vi "Test Timed Door API.vi"() -> ()   [LabVIEW 2018]
uses:
  Timed Door.lvclass
  Door/Door.lvclass
  Timed Door.lvclass/Timed Door.ctl
  Set Door.vi
  Set Target Time (seconds).vi
panel:
  out "error out":errorcluster
  in  "Timed Door Target Time (seconds)":dbl=5.0
  in  "Door Switch":enum32{"Open Door", "Close Door"}(radio)=enum."Close Door"
  out "Door":u16(ring)
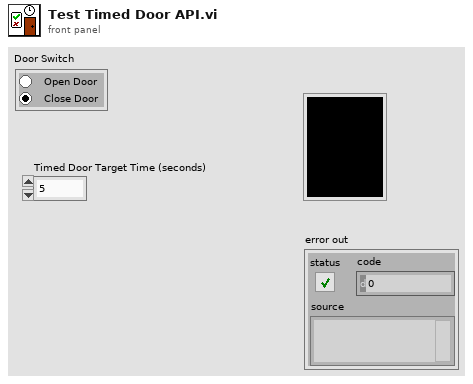
[diagram p1: front panel]
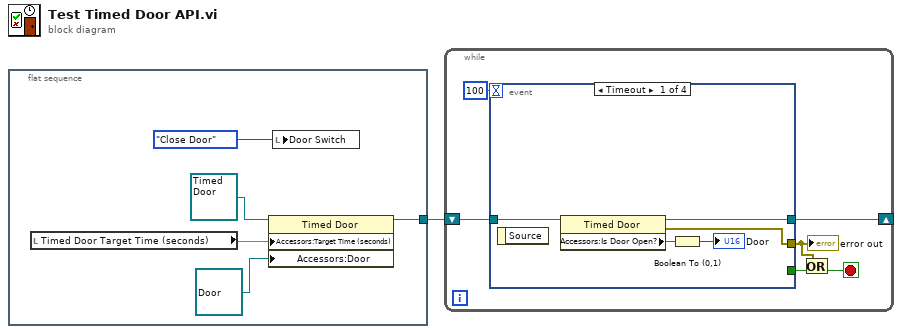
[diagram p0: block diagram]
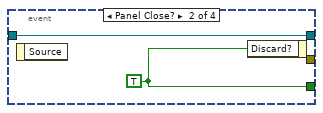
[diagram p2: hidden frame]
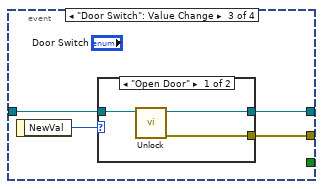
[diagram p3: hidden frame]
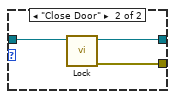
[diagram p4: hidden frame]
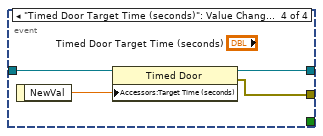
[diagram p5: hidden frame]
diagram:
  n1 = flat-sequence {
    tunnel: [w4] -> w1
    frame #0 {
      n2 = local read "Timed Door Target Time (seconds)"() -> (w5:dbl)
      n3 = property class="Timed Door"(reference=refnum<class "Timed Door.lvclass"> refnum ("Timed Door.lvclass"), "Accessors:Target Time (seconds)"=w5, "Accessors:Door"=refnum<class "Door.lvclass"> refnum ("Door")) -> (reference out=w4:refnum<class "Timed Door.lvclass">)  [unwired: 1 in, 1 out]
      n4 = local write "Door Switch"(enum32{"Open Door", "Close Door"}."Close Door" ("Door Switch")) -> ()
    }
  }
  n5 = while {
    shift-right: [w9] -> _
    shift-left: w1 -> [w11]
    stop <- w8 stop-if-true
    n6 = event shown="[0] Timeout" {
      selector: _ -> [_ _ _ _]
      dyn-events: _ -> [_ _ _ _]
      timeout: 100 -> [_ _ _ _]
      tunnel: w11 -> [w14 w18 w23 w31]
      tunnel: [_ w19 _ _] -> w10
      tunnel: [w15 w18 w22 w33] -> w9
      tunnel: [w13 _ w20 w30] -> w7
      event Timeout {
        n7 = event-data() -> ()  [unwired: 1 in, 1 out]
        n8 = property class="Timed Door"(reference=w14) -> (reference out=w15:refnum<class "Timed Door.lvclass">, error out=w13:errorcluster, "Accessors:Is Door Open?"=w17:bool)  [unwired: 1 in]
        n9 = Boolean To (0,1)(Boolean=w17) -> (0, 1=→"Door":i16)
      }
      event Panel Close? {
        w19 = TRUE ("Discard?")
        n10 = event-data() -> ()  [unwired: 1 in, 1 out]
        n11 = event-data("Discard?"=w19) -> ()  [unwired: 1 in, 1 out]
      }
      event "Door Switch": Value Change {
        n12 = event-data() -> ("NewVal"=w21:enum32{"Open Door", "Close Door"})  [unwired: 1 in]
        n13 = case shown="\"Open Door\"" w21 {
          tunnel: w23 -> [w26 w29]
          tunnel: [w25 w28] -> w22
          tunnel: [w24 w27] -> w20
          frame "Open Door" {
            n14 = call-dynamic "Unlock.vi"("Timed Door in"=w26) -> ("error out"=w24:errorcluster, "Timed Door out"=w25:refnum<class "Timed Door.lvclass">)  [unwired: 9 in]
          }
          frame "Close Door" {
            n15 = call-dynamic "Lock.vi"("Timed Door in"=w29) -> ("error out"=w27:errorcluster, "Timed Door out"=w28:refnum<class "Timed Door.lvclass">)  [unwired: 9 in]
          }
        }
      }
      event "Timed Door Target Time (seconds)": Value Change {
        n16 = event-data() -> ("NewVal"=w32:dbl)  [unwired: 1 in]
        n17 = property class="Timed Door"(reference=w31, "Accessors:Target Time (seconds)"=w32) -> (reference out=w33:refnum<class "Timed Door.lvclass">, error out=w30:errorcluster)  [unwired: 1 in]
      }
    }
    "error out" <- w7
    n18 = Or(x=w7, y=w10) -> (x .or. y?=w8:bool)
  }
